vi "Dropdown - global.vi"(0 "Engine Mode In":T1(ring), 1 "AbbrS In":string[](array[string]), 2 "Ring Index In":u16, 3 "Left In":i16, 4 "Top In":i16, 5 "Abbr In":string, 6 "Cursor Pos In":i32[](array[numeric]), 7 "Error In":errorcluster, 8 "Global Mode":T2(ring)) -> (11 "Engine Started":bool, 12 "Cursor Pos Out":i32[](array[numeric]), 13 "Error Out":errorcluster, 14 "Engine Mode Out":T1(ring), 15 "AbbrS Out":string[](array[string]), 16 "Ring Index Out":u16, 17 "Left Out":i16, 18 "Top Out":i16, 19 "Abbr Out":string="DNE")   [LabVIEW 2019]
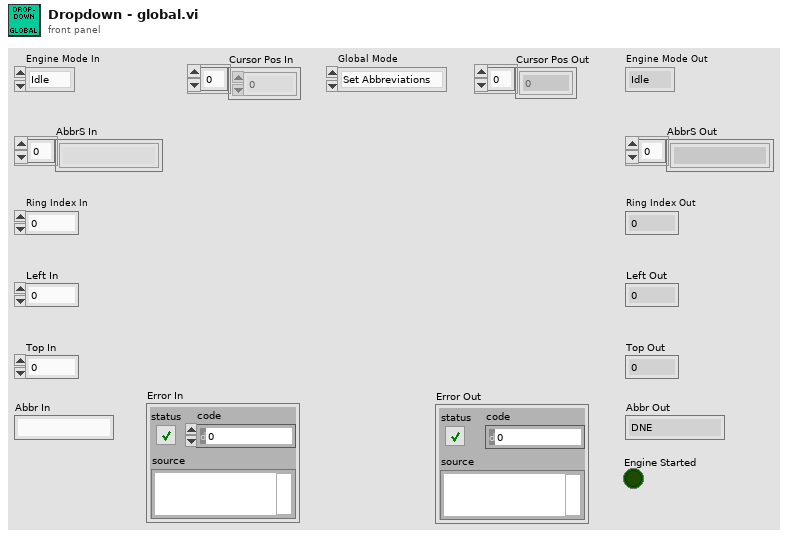
[diagram p1: front panel]
types:
  T1 = enum16{"Idle", "Reveal Dropdown", "Hide FP", "Set Options", "Close Program"}
  T2 = enum16{"Set Abbreviations", "Set Engine Mode", "Set Enum Position", "Get Abbreviation", "Write Abbreviation", "Read Enum Position", "Read Engine Mode", "Read Abbreviations", "Engine Started", "Check Engine", "Init Global", "Set Cursor", "Read Cursor"}
  T3 = enum16{"Idle", "Reveal Dropdown", "Hide FP", "Set Options"}
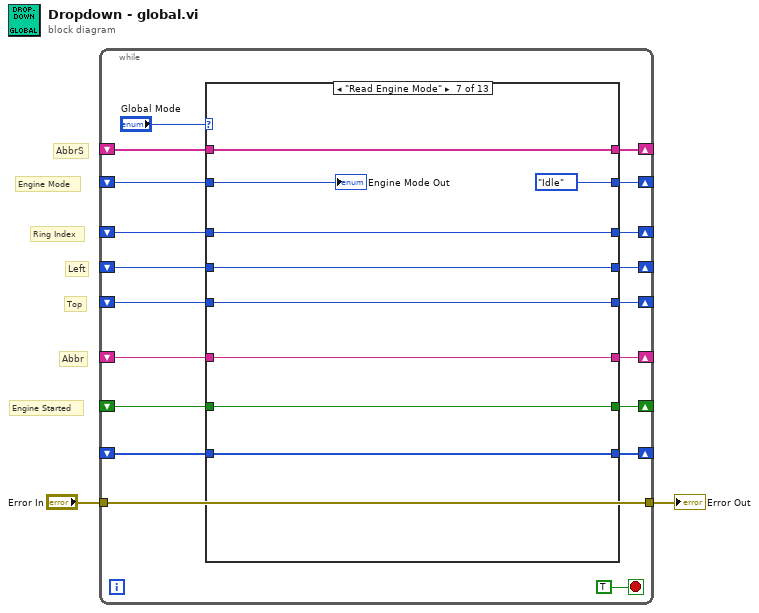
[diagram p0: block diagram]
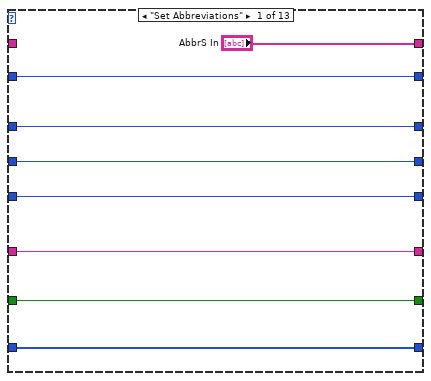
[diagram p2: hidden frame]
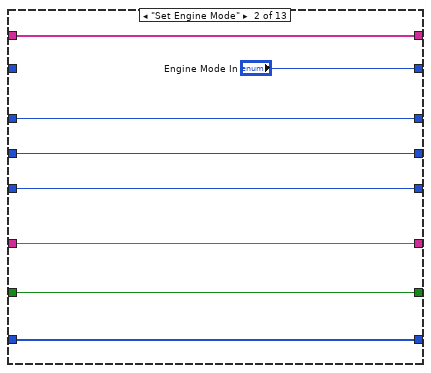
[diagram p3: hidden frame]
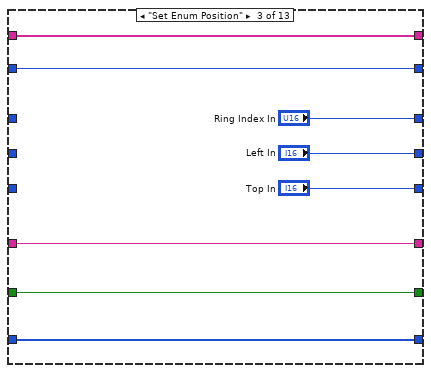
[diagram p4: hidden frame]
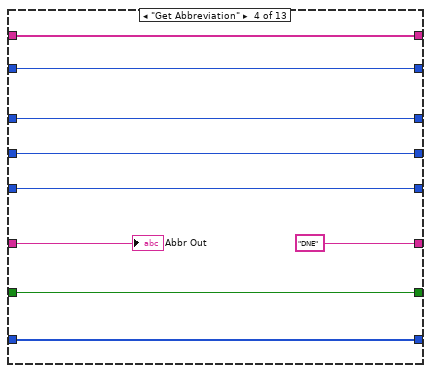
[diagram p5: hidden frame]
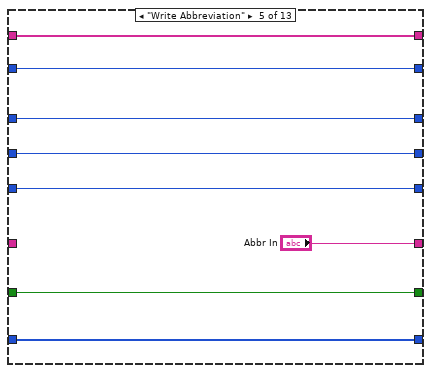
[diagram p6: hidden frame]
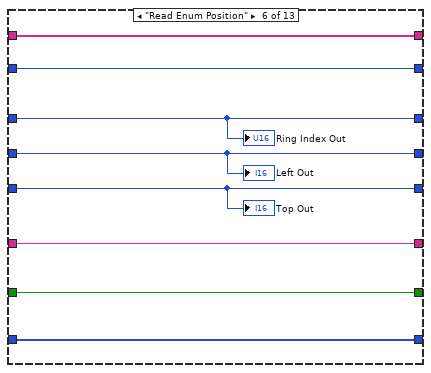
[diagram p7: hidden frame]
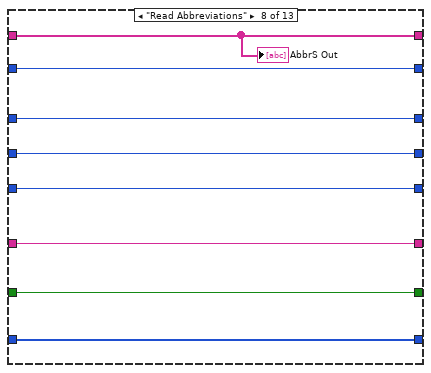
[diagram p8: hidden frame]
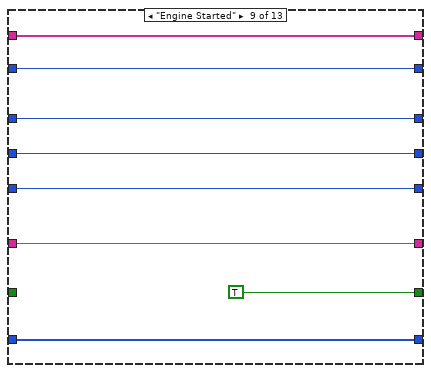
[diagram p9: hidden frame]
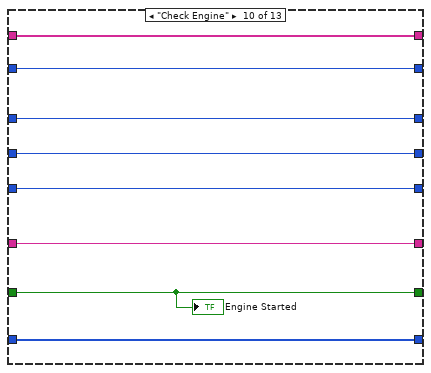
[diagram p10: hidden frame]
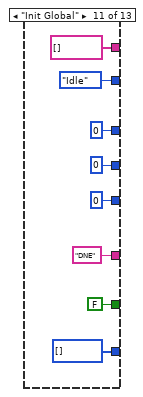
[diagram p11: hidden frame]
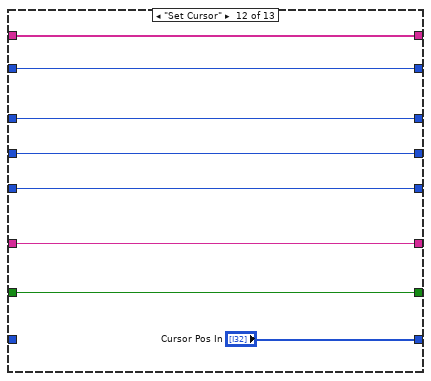
[diagram p12: hidden frame]
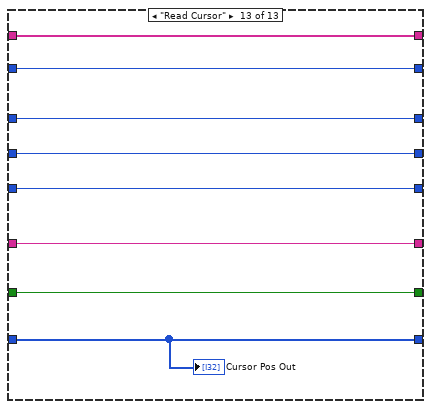
[diagram p13: hidden frame]
diagram:
  # "Engine Started"
  # "Abbr"
  # "Top"
  # "Left"
  # "Ring Index"
  # "AbbrS"
  # "Engine Mode"
  n1 = while {
    shift-right: [w20] -> _
    shift-left: _ -> [w19]
    shift-right: [w18] -> _
    shift-left: _ -> [w17]
    shift-right: [w16] -> _
    shift-left: _ -> [w13]
    shift-right: [w15] -> _
    shift-left: _ -> [w12]
    shift-right: [w14] -> _
    shift-left: _ -> [w11]
    shift-right: [w10] -> _
    shift-left: _ -> [w9]
    tunnel: [w8] -> w2
    tunnel: "Error In" -> [w8]
    shift-right: [w6] -> _
    shift-left: _ -> [w5]
    shift-right: [w4] -> _
    shift-left: _ -> [w3]
    stop <- TRUE stop-if-true
    n2 = case shown="\"Read Engine Mode\"" "Global Mode" {
      tunnel: ["AbbrS In" w37 w42 w49 w57 w70 w79 w87 w94 w103 string[] [] ("AbbrS In") w119 w120] -> w20
      tunnel: w19 -> [_ w37 w42 w49 w57 w70 w79 w87 w94 w103 _ w119 w120]
      tunnel: [w28 "Engine Mode In" w41 w50 w58 w69 T1."Idle" ("Mode") w86 w93 w102 T3."Idle" ("Engine Mode In") w118 w121] -> w18
      tunnel: w17 -> [w28 _ w41 w50 w58 w69 w72 w86 w93 w102 _ w118 w121]
      tunnel: [w27 w36 "Ring Index In" w51 w59 w68 w78 w85 w92 w101 u16 0 ("Ring Index In") w117 w122] -> w16
      tunnel: [w26 w35 "Left In" w52 w60 w67 w77 w84 w91 w100 i16 0 ("Left In") w116 w123] -> w15
      tunnel: [w25 w34 "Top In" w53 w61 w66 w76 w83 w90 w99 i16 0 ("Top In") w115 w124] -> w14
      tunnel: w13 -> [w27 w36 _ w51 w59 w68 w78 w85 w92 w101 _ w117 w122]
      tunnel: w12 -> [w26 w35 _ w52 w60 w67 w77 w84 w91 w100 _ w116 w123]
      tunnel: w11 -> [w25 w34 _ w53 w61 w66 w76 w83 w90 w99 _ w115 w124]
      tunnel: [w23 w33 w40 "DNE" ("Abbr In") "Abbr In" w65 w75 w82 w89 w98 "DNE" ("Abbr In") w114 w125] -> w10
      tunnel: w9 -> [w23 w33 w40 w54 _ w65 w75 w82 w89 w98 _ w114 w125]
      tunnel: [w24 w32 w39 w47 w56 w64 w74 w81 TRUE w97 FALSE w113 w126] -> w6
      tunnel: w5 -> [w24 w32 w39 w47 w56 w64 w74 w81 _ w97 _ w113 w126]
      tunnel: [w22 w31 w38 w46 w55 w63 w73 w80 w88 w96 i32[] [] ("Cursor Pos In") "Cursor Pos In" w127] -> w4
      tunnel: w3 -> [w22 w31 w38 w46 w55 w63 w73 w80 w88 w96 _ _ w127]
      frame "Set Abbreviations" {
      }
      frame "Set Engine Mode" {
      }
      frame "Set Enum Position" {
      }
      frame "Get Abbreviation" {
        "Abbr Out" <- w54
      }
      frame "Write Abbreviation" {
      }
      frame "Read Enum Position" {
        "Top Out" <- w66
        "Left Out" <- w67
        "Ring Index Out" <- w68
      }
      frame "Read Engine Mode" {
        "Engine Mode Out" <- w72
      }
      frame "Read Abbreviations" {
        "AbbrS Out" <- w87
      }
      frame "Engine Started" {
      }
      frame "Check Engine" {
        "Engine Started" <- w97
      }
      frame "Init Global" {
      }
      frame "Set Cursor" {
      }
      frame "Read Cursor" {
        "Cursor Pos Out" <- w127
      }
    }
  }
  "Error Out" <- w2
